vi "GetTerms4.vi"(0 "XRef":T12, 1 "State In":T10) -> (14 "Terms":T2, 15 "Fatal Error Out":T1)   [LabVIEW 2015, in "LVJSON.lvlib" / "Get Object Parameters.xnode"]
uses:
  Get Object Parameters.xnode
  <vilib>/XNodeSupport/XNodeXNodeRef.ctl
  State.ctl
  Parameter.ctl
  <vilib>/XNodeSupport/XNodeTerm4Array.ctl
  <vilib>/XNodeSupport/XNodeTerm4.ctl
  <vilib>/XNodeSupport/XNodeString.ctl
  <vilib>/XNodeSupport/XNodeVariant.ctl
  <vilib>/XNodeSupport/XNodeRect32.ctl
  <vilib>/XNodeSupport/XNodeInt.ctl
  <vilib>/XNodeSupport/XNodeBool.ctl
  <vilib>/XNodeSupport/XNodeTermDirection.ctl
  <vilib>/XNodeSupport/XNodeErrorCluster.ctl
  JSON Object.lvclass
  JSON Numeric/JSON Numeric.lvclass
  JSON String/JSON String.lvclass
  JSON Boolean/JSON Boolean.lvclass
  JSON Datatype/JSON Null.lvclass
  JSON Array/JSON Array.lvclass
  offsets.vi
  <vilib>/XNodeSupport/NI_XNodeSupport.lvlib
  Shared/Shared.lvlib
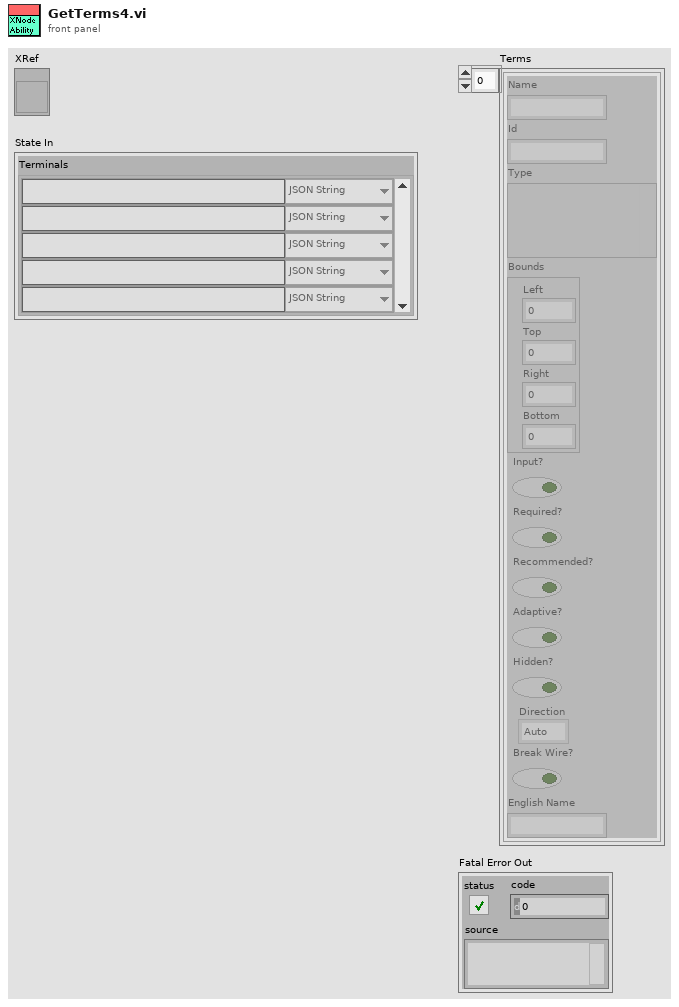
[diagram p1: front panel]
types:
  T1 = typedef "NI_XNodeSupport.lvlib/XNodeErrorCluster.ctl" = errorcluster
  T2 = typedef "NI_XNodeSupport.lvlib/XNodeTerm4Array.ctl" = T3[]
  T3 = typedef "NI_XNodeSupport.lvlib/XNodeTerm4.ctl" = cluster{"Name":T4, "Id":T4, "Type":T5, "Bounds":T6, "Input?":T8, "Required?":T8, "Recommended?":T8, "Adaptive?":T8, "Hidden?":T8, "Direction":T9, "Break Wire?":T8, "English Name":T4}
  T4 = typedef "NI_XNodeSupport.lvlib/XNodeString.ctl" = string
  T5 = typedef "NI_XNodeSupport.lvlib/XNodeVariant.ctl" = variant
  T6 = typedef "NI_XNodeSupport.lvlib/XNodeRect32.ctl" = cluster{"Left":T7, "Top":T7, "Right":T7, "Bottom":T7}
  T7 = typedef "NI_XNodeSupport.lvlib/XNodeInt.ctl" = i32
  T8 = typedef "NI_XNodeSupport.lvlib/XNodeBool.ctl" = bool
  T9 = typedef "NI_XNodeSupport.lvlib/XNodeTermDirection.ctl" = enum32{"Auto", "Up", "Down", "Left", "Right", "Center"}
  T10 = typedef "LVJSON.lvlib/Get Object Parameters.xnode/State.ctl" = cluster{"Terminals":T11[]}
  T11 = typedef "LVJSON.lvlib/Shared.lvlib/Parameter.ctl" = cluster{"Parameter Name":string, "JSON Type":enum16{"JSON String", "JSON Numeric", "JSON Boolean", "JSON", "JSON Object", "JSON Array", "String Value", "Numeric Value", "Boolean Value"}}
  T12 = typedef "NI_XNodeSupport.lvlib/XNodeXNodeRef.ctl" = refnum<vi>
  T13 = enum16{"JSON String", "JSON Numeric", "JSON Boolean", "JSON", "JSON Object", "JSON Array", "String Value", "Numeric Value", "Boolean Value"}
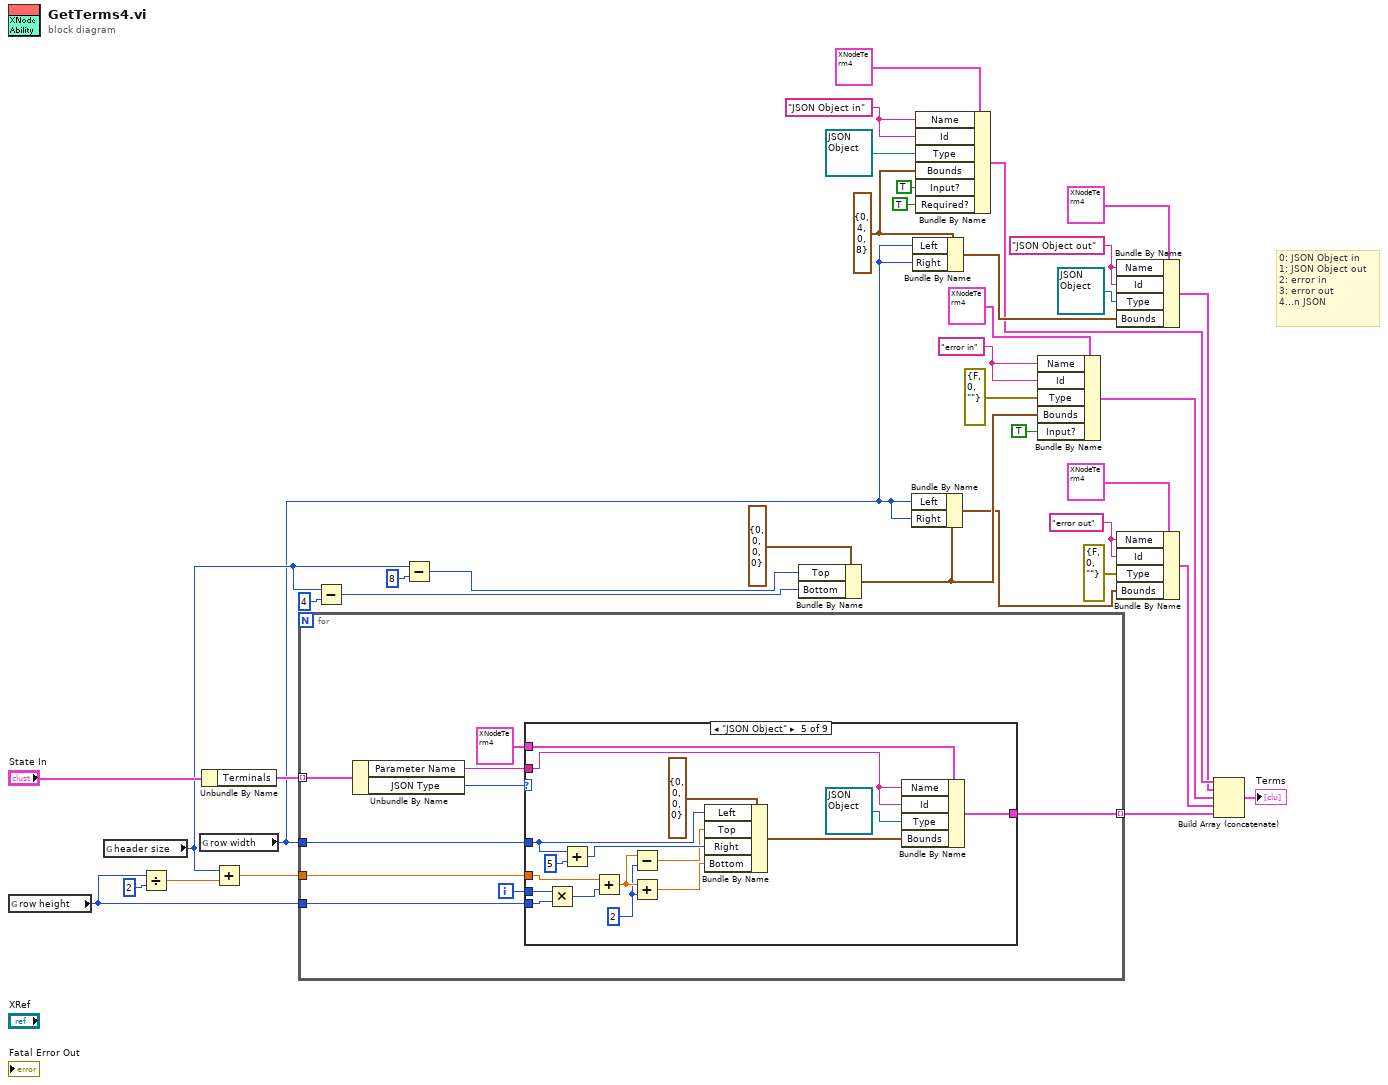
[diagram p0: block diagram]
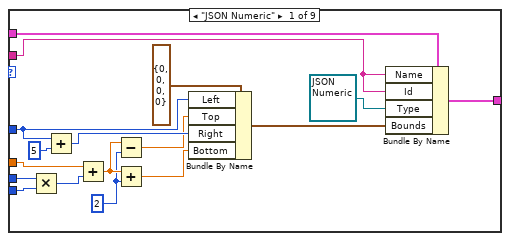
[diagram p2: hidden frame]
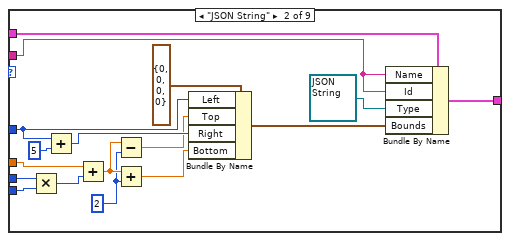
[diagram p3: hidden frame]
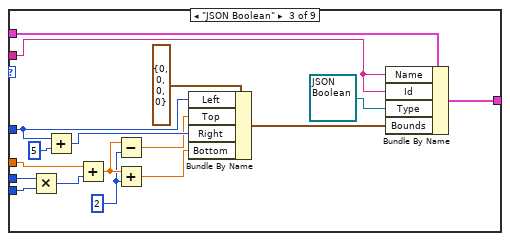
[diagram p4: hidden frame]
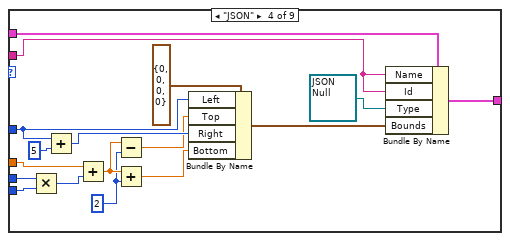
[diagram p5: hidden frame]
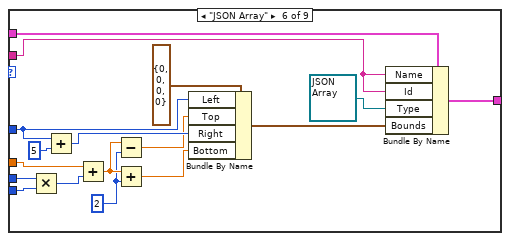
[diagram p6: hidden frame]
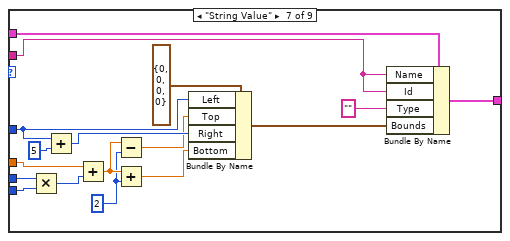
[diagram p7: hidden frame]
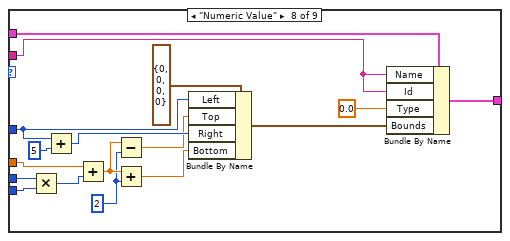
[diagram p8: hidden frame]
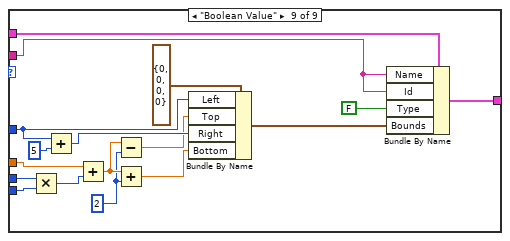
[diagram p9: hidden frame]
diagram:
  w9 = T4 "JSON Object out" ("Name")
  w5 = T6 {"Left"=0, "Top"=4, "Right"=0, "Bottom"=8} ("Bounds")
  w16 = T4 "JSON Object in" ("Name")
  w28 = T4 "error out" ("Name")
  w31 = T4 "error in" ("Name")
  # "0: JSON Object in\n1: JSON Object out\n2: error in\n3: error out\n4...n JSON"
  n1 = global read "offsets.vi" "row height"() -> (w36:i16)
  n2 = global read "offsets.vi" "header size"() -> (w25:i16)
  n3 = Divide(x=w36, y=i16 2) -> (x/y=w34:dbl)
  n4 = global read "offsets.vi" "row width"() -> (w6:i16)
  n5 = Unbundle By Name("State In") -> ("Terminals"=w37:T11[])
  n6 = Add(x=w25, y=w34) -> (x+y=w33:dbl)
  n7 = for {
    tunnel: w37 -> [w46] mode=indexing
    tunnel: w36 -> [w42]
    tunnel: w33 -> [w43]
    tunnel: w6 -> [w40]
    tunnel: [w39] -> w13 mode=indexing
    i -> [w41]
    n8 = Unbundle By Name(w46) -> ("Parameter Name"=w45:string, "JSON Type"=w44:T13)
    n9 = case shown="\"JSON Object\"" w44 {
      tunnel: T3 {"Name"="", "Id"="", "Type"=variant, "Bounds"={"Left"=0, "Top"=0, "Right"=0, "Bottom"=0}, "Input?"=FALSE, "Required?"=FALSE, "Recommended?"=FALSE, "Adaptive?"=FALSE, "Hidden?"=FALSE, "Direction"=enum."Auto", "Break Wire?"=FALSE, "English Name"=""} ("Term 4") -> [w64 w81 w98 w115 w132 w149 w166 w183 w200]
      tunnel: w45 -> [w51 w68 w85 w102 w119 w136 w154 w171 w188]
      tunnel: [w62 w79 w96 w113 w130 w147 w165 w182 w199] -> w39
      tunnel: w43 -> [w57 w74 w91 w108 w125 w142 w160 w177 w194]
      tunnel: w42 -> [w60 w77 w94 w111 w128 w145 w163 w180 w197]
      tunnel: w41 -> [w59 w76 w93 w110 w127 w144 w162 w179 w196]
      tunnel: w40 -> [w53 w70 w87 w104 w121 w138 w156 w173 w190]
      frame "JSON Numeric" {
        w49 = T7 2 ("Right")
        n10 = Multiply(x=w59, y=w60) -> (x*y=w58:i32)
        n11 = Add(x=w53, y=T7 5 ("Right")) -> (x+y=w52:T7)
        n12 = Add(x=w57, y=w58) -> (x+y=w50:dbl)
        n13 = Subtract(x=w50, y=w49) -> (x-y=w48:dbl)
        n14 = Add(x=w50, y=w49) -> (x+y=w56:dbl)
        n15 = Bundle By Name(cluster=T6 {"Left"=0, "Top"=0, "Right"=0, "Bottom"=0} ("Bounds"), "Left"=w53, "Top"=w48, "Right"=w52, "Bottom"=w56) -> (w55:T6)
        n16 = Bundle By Name(cluster=w64, "Name"=w51, "Id"=w51, "Type"=refnum<class "JSON Numeric.lvclass"> refnum ("JSON String out"), "Bounds"=w55) -> (w62:T3)
      }
      frame "JSON String" {
        w66 = T7 2 ("Right")
        n17 = Multiply(x=w76, y=w77) -> (x*y=w75:i32)
        n18 = Add(x=w70, y=T7 5 ("Right")) -> (x+y=w69:T7)
        n19 = Add(x=w74, y=w75) -> (x+y=w67:dbl)
        n20 = Subtract(x=w67, y=w66) -> (x-y=w65:dbl)
        n21 = Add(x=w67, y=w66) -> (x+y=w73:dbl)
        n22 = Bundle By Name(cluster=T6 {"Left"=0, "Top"=0, "Right"=0, "Bottom"=0} ("Bounds"), "Left"=w70, "Top"=w65, "Right"=w69, "Bottom"=w73) -> (w72:T6)
        n23 = Bundle By Name(cluster=w81, "Name"=w68, "Id"=w68, "Type"=refnum<class "JSON String.lvclass"> refnum ("JSON String out"), "Bounds"=w72) -> (w79:T3)
      }
      frame "JSON Boolean" {
        w83 = T7 2 ("Right")
        n24 = Multiply(x=w93, y=w94) -> (x*y=w92:i32)
        n25 = Add(x=w87, y=T7 5 ("Right")) -> (x+y=w86:T7)
        n26 = Add(x=w91, y=w92) -> (x+y=w84:dbl)
        n27 = Subtract(x=w84, y=w83) -> (x-y=w82:dbl)
        n28 = Add(x=w84, y=w83) -> (x+y=w90:dbl)
        n29 = Bundle By Name(cluster=T6 {"Left"=0, "Top"=0, "Right"=0, "Bottom"=0} ("Bounds"), "Left"=w87, "Top"=w82, "Right"=w86, "Bottom"=w90) -> (w89:T6)
        n30 = Bundle By Name(cluster=w98, "Name"=w85, "Id"=w85, "Type"=refnum<class "JSON Boolean.lvclass"> refnum ("JSON String out"), "Bounds"=w89) -> (w96:T3)
      }
      frame "JSON" {
        w100 = T7 2 ("Right")
        n31 = Multiply(x=w110, y=w111) -> (x*y=w109:i32)
        n32 = Add(x=w104, y=T7 5 ("Right")) -> (x+y=w103:T7)
        n33 = Add(x=w108, y=w109) -> (x+y=w101:dbl)
        n34 = Subtract(x=w101, y=w100) -> (x-y=w99:dbl)
        n35 = Add(x=w101, y=w100) -> (x+y=w107:dbl)
        n36 = Bundle By Name(cluster=T6 {"Left"=0, "Top"=0, "Right"=0, "Bottom"=0} ("Bounds"), "Left"=w104, "Top"=w99, "Right"=w103, "Bottom"=w107) -> (w106:T6)
        n37 = Bundle By Name(cluster=w115, "Name"=w102, "Id"=w102, "Type"=refnum<class "JSON Null.lvclass"> refnum ("JSON String out"), "Bounds"=w106) -> (w113:T3)
      }
      frame "JSON Object" {
        w117 = T7 2 ("Right")
        n38 = Multiply(x=w127, y=w128) -> (x*y=w126:i32)
        n39 = Add(x=w121, y=T7 5 ("Right")) -> (x+y=w120:T7)
        n40 = Add(x=w125, y=w126) -> (x+y=w118:dbl)
        n41 = Subtract(x=w118, y=w117) -> (x-y=w116:dbl)
        n42 = Add(x=w118, y=w117) -> (x+y=w124:dbl)
        n43 = Bundle By Name(cluster=T6 {"Left"=0, "Top"=0, "Right"=0, "Bottom"=0} ("Bounds"), "Left"=w121, "Top"=w116, "Right"=w120, "Bottom"=w124) -> (w123:T6)
        n44 = Bundle By Name(cluster=w132, "Name"=w119, "Id"=w119, "Type"=refnum<class "JSON Object.lvclass"> refnum ("JSON String out"), "Bounds"=w123) -> (w130:T3)
      }
      frame "JSON Array" {
        w134 = T7 2 ("Right")
        n45 = Multiply(x=w144, y=w145) -> (x*y=w143:i32)
        n46 = Add(x=w138, y=T7 5 ("Right")) -> (x+y=w137:T7)
        n47 = Add(x=w142, y=w143) -> (x+y=w135:dbl)
        n48 = Subtract(x=w135, y=w134) -> (x-y=w133:dbl)
        n49 = Add(x=w135, y=w134) -> (x+y=w141:dbl)
        n50 = Bundle By Name(cluster=T6 {"Left"=0, "Top"=0, "Right"=0, "Bottom"=0} ("Bounds"), "Left"=w138, "Top"=w133, "Right"=w137, "Bottom"=w141) -> (w140:T6)
        n51 = Bundle By Name(cluster=w149, "Name"=w136, "Id"=w136, "Type"=refnum<class "JSON Array.lvclass"> refnum ("JSON String out"), "Bounds"=w140) -> (w147:T3)
      }
      frame "String Value" {
        w152 = T7 2 ("Right")
        n52 = Multiply(x=w162, y=w163) -> (x*y=w161:i32)
        n53 = Add(x=w156, y=T7 5 ("Right")) -> (x+y=w155:T7)
        n54 = Add(x=w160, y=w161) -> (x+y=w153:dbl)
        n55 = Subtract(x=w153, y=w152) -> (x-y=w151:dbl)
        n56 = Add(x=w153, y=w152) -> (x+y=w159:dbl)
        n57 = Bundle By Name(cluster=T6 {"Left"=0, "Top"=0, "Right"=0, "Bottom"=0} ("Bounds"), "Left"=w156, "Top"=w151, "Right"=w155, "Bottom"=w159) -> (w158:T6)
        n58 = Bundle By Name(cluster=w166, "Name"=w154, "Id"=w154, "Type"="", "Bounds"=w158) -> (w165:T3)
      }
      frame "Numeric Value" {
        w169 = T7 2 ("Right")
        n59 = Multiply(x=w179, y=w180) -> (x*y=w178:i32)
        n60 = Add(x=w173, y=T7 5 ("Right")) -> (x+y=w172:T7)
        n61 = Add(x=w177, y=w178) -> (x+y=w170:dbl)
        n62 = Subtract(x=w170, y=w169) -> (x-y=w168:dbl)
        n63 = Add(x=w170, y=w169) -> (x+y=w176:dbl)
        n64 = Bundle By Name(cluster=T6 {"Left"=0, "Top"=0, "Right"=0, "Bottom"=0} ("Bounds"), "Left"=w173, "Top"=w168, "Right"=w172, "Bottom"=w176) -> (w175:T6)
        n65 = Bundle By Name(cluster=w183, "Name"=w171, "Id"=w171, "Type"=0.0, "Bounds"=w175) -> (w182:T3)
      }
      frame "Boolean Value" {
        w186 = T7 2 ("Right")
        n66 = Multiply(x=w196, y=w197) -> (x*y=w195:i32)
        n67 = Add(x=w190, y=T7 5 ("Right")) -> (x+y=w189:T7)
        n68 = Add(x=w194, y=w195) -> (x+y=w187:dbl)
        n69 = Subtract(x=w187, y=w186) -> (x-y=w185:dbl)
        n70 = Add(x=w187, y=w186) -> (x+y=w193:dbl)
        n71 = Bundle By Name(cluster=T6 {"Left"=0, "Top"=0, "Right"=0, "Bottom"=0} ("Bounds"), "Left"=w190, "Top"=w185, "Right"=w189, "Bottom"=w193) -> (w192:T6)
        n72 = Bundle By Name(cluster=w200, "Name"=w188, "Id"=w188, "Type"=FALSE, "Bounds"=w192) -> (w199:T3)
      }
    }
  }
  n73 = Subtract(x=w25, y=i16 4) -> (x-y=w22:i16)
  n74 = Subtract(x=w25, y=i16 8) -> (x-y=w21:i16)
  n75 = Bundle By Name(cluster=T6 {"Left"=0, "Top"=0, "Right"=0, "Bottom"=0} ("Bounds"), "Top"=w21, "Bottom"=w22) -> (w20:T6)
  n76 = Bundle By Name(cluster=w20, "Left"=w6, "Right"=w6) -> (w19:T6)
  n77 = Bundle By Name(cluster=w5, "Left"=w6, "Right"=w6) -> (w4:T6)
  n78 = Bundle By Name(cluster=T3 {"Name"="", "Id"="", "Type"=variant, "Bounds"={"Left"=0, "Top"=0, "Right"=0, "Bottom"=0}, "Input?"=FALSE, "Required?"=FALSE, "Recommended?"=FALSE, "Adaptive?"=FALSE, "Hidden?"=FALSE, "Direction"=enum."Auto", "Break Wire?"=FALSE, "English Name"=""} ("Term 4"), "Name"=w16, "Id"=w16, "Type"=refnum<class "JSON Object.lvclass"> refnum ("JSON String out"), "Bounds"=w5, "Input?"=T8 TRUE, "Required?"=T8 TRUE) -> (w3:T3)
  n79 = Bundle By Name(cluster=T3 {"Name"="", "Id"="", "Type"=variant, "Bounds"={"Left"=0, "Top"=0, "Right"=0, "Bottom"=0}, "Input?"=FALSE, "Required?"=FALSE, "Recommended?"=FALSE, "Adaptive?"=FALSE, "Hidden?"=FALSE, "Direction"=enum."Auto", "Break Wire?"=FALSE, "English Name"=""} ("Term 4"), "Name"=w31, "Id"=w31, "Type"=errorcluster {"status"=FALSE, "code"=0, "source"=""} ("error constant"), "Bounds"=w20, "Input?"=T8 TRUE) -> (w18:T3)
  n80 = Bundle By Name(cluster=T3 {"Name"="", "Id"="", "Type"=variant, "Bounds"={"Left"=0, "Top"=0, "Right"=0, "Bottom"=0}, "Input?"=FALSE, "Required?"=FALSE, "Recommended?"=FALSE, "Adaptive?"=FALSE, "Hidden?"=FALSE, "Direction"=enum."Auto", "Break Wire?"=FALSE, "English Name"=""} ("Term 4"), "Name"=w9, "Id"=w9, "Type"=refnum<class "JSON Object.lvclass"> refnum ("JSON String out"), "Bounds"=w4) -> (w2:T3)
  n81 = Bundle By Name(cluster=T3 {"Name"="", "Id"="", "Type"=variant, "Bounds"={"Left"=0, "Top"=0, "Right"=0, "Bottom"=0}, "Input?"=FALSE, "Required?"=FALSE, "Recommended?"=FALSE, "Adaptive?"=FALSE, "Hidden?"=FALSE, "Direction"=enum."Auto", "Break Wire?"=FALSE, "English Name"=""} ("Term 4"), "Name"=w28, "Id"=w28, "Type"=errorcluster {"status"=FALSE, "code"=0, "source"=""} ("error constant"), "Bounds"=w19) -> (w17:T3)
  n82 = Build Array (concatenate)(w3, w2, w18, w17, w13) -> (→"Terms":T3[])
